vi "Array1DMean.vi"(11 "Array":dbl[](array[numeric])) -> (3 "Numeric Control":dbl)   [LabVIEW 2014]
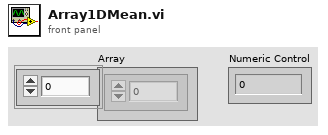
[diagram p1: front panel]
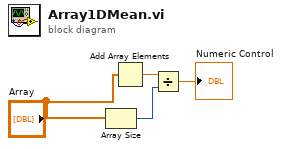
[diagram p0: block diagram]
diagram:
  n1 = Array Size(array="Array") -> (size(s)=w3:i32)
  n2 = Add Array Elements(numeric array="Array") -> (sum=w2:dbl)
  n3 = Divide(x=w2, y=w3) -> (x/y=→"Numeric Control":dbl)
